vi "Read Props.vi"(8 "error in (no error)":errorcluster, 11 "NumRangeBoolEditorPanel in":refnum<class "NumRangeBoolEditorPanel.lvclass">) -> (0 "error out":errorcluster, 2 "Props":T1, 3 "NumRangeBoolEditorPanel out":refnum<class "NumRangeBoolEditorPanel.lvclass">)   [LabVIEW 2020, in "VolatusGUIControls.lvlib" / "NumRangeBoolEditorPanel.lvclass"]
uses:
  NumRangeBoolEditorPanel.lvclass
  NumRangeBoolEditorPanel.lvclass/NumRangeBoolEditorPanel.ctl
  JSON Props.ctl
  VolatusGUIEditorCore/Label Props.ctl
  VolatusGUIEditorCore/VolatusGUIEditorCore.lvlib
  VolatusGUIEditorCore/Position Props.ctl
  VolatusGUIEditorCore/Boolean Color Props.ctl
  Props.ctl
  VolatusGUIControls.lvlib
  68272f9f-15cf-44f9-b6ab-6d8c4d3063f4.vi
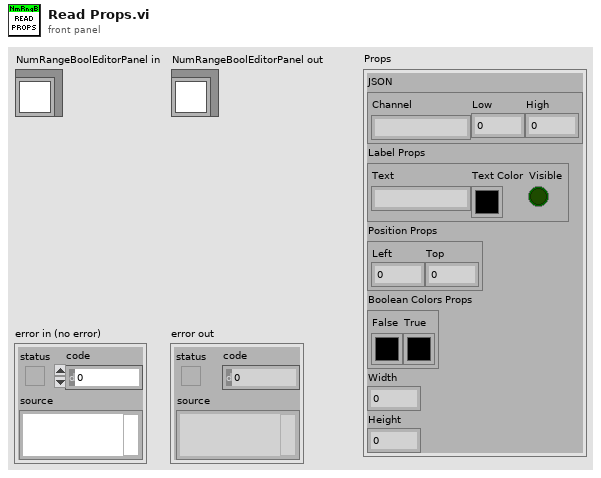
[diagram p1: front panel]
types:
  T1 = typedef "VolatusGUIControls.lvlib/NumRangeBoolEditorPanel.lvclass/Props.ctl" = cluster{"JSON":T2, "Label Props":T3, "Position Props":T4, "Boolean Colors Props":T5, "Width":u16, "Height":u16}
  T2 = typedef "VolatusGUIControls.lvlib/NumRangeBoolEditorPanel.lvclass/JSON Props.ctl" = cluster{"Channel":string, "Low":dbl, "High":dbl}
  T3 = typedef "VolatusGUIEditorCore.lvlib/Label Props.ctl" = cluster{"Text":string, "Text Color":u32, "Visible":bool}
  T4 = typedef "VolatusGUIEditorCore.lvlib/Position Props.ctl" = cluster{"Left":i32, "Top":i32}
  T5 = typedef "VolatusGUIEditorCore.lvlib/Boolean Color Props.ctl" = cluster{"False":u32, "True":u32}
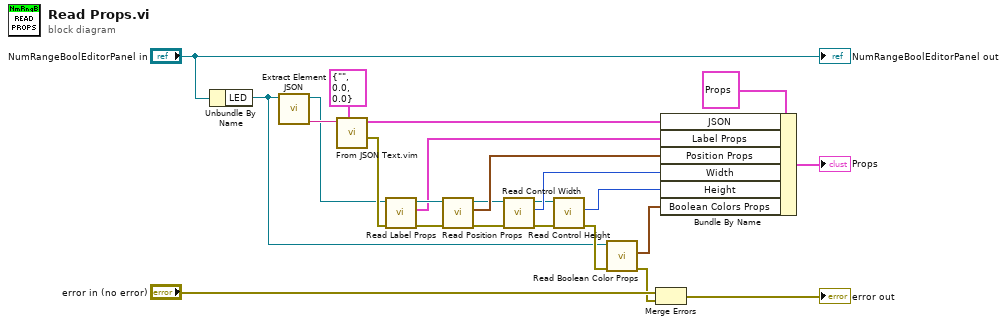
[diagram p0: block diagram]
diagram:
  n1 = Unbundle By Name("NumRangeBoolEditorPanel in") -> ("LED"=w4:refnum<vi>)
  n2 = call "Extract Element JSON.vi"("Ctl Refnum in"=w4) -> ("JSON"=w20:string, "Ctl Refnum"=w16:refnum<vi>)  [unwired: 7 in, 2 out]
  n3 = call "From JSON Text.vim"("Data Type and Default Value"=T2 {"Channel"="", "Low"=0.0, "High"=0.0} ("JSON"), "JSON"=w20) -> ("error out"=w24:errorcluster, "Data out"=w17:T2)  [unwired: 8 in]
  n4 = call "Read Label Props.vi"("error in (no error)"=w24, "Ctl Refnum in"=w16) -> ("error out"=w15:errorcluster, "Label Props"=w13:T3, "Ctl Refnum"=w14:refnum<vi>)  [unwired: 7 in]
  n5 = call "Read Position Props.vi"("error in (no error)"=w15, "Ctl Refnum in"=w14) -> ("error out"=w11:errorcluster, "Position Props"=w12:T4, "Ctl Refnum"=w10:refnum<vi>)  [unwired: 7 in]
  n6 = call "Read Control Width.vi"("error in"=w11, "Control in"=w10) -> ("error out"=w8:errorcluster, "Width"=w9:u32, "Control"=w7:refnum<vi>)  [unwired: 7 in]
  n7 = call "Read Control Height.vi"("error in"=w8, "Control in"=w7) -> ("error out"=w5:errorcluster, "Height"=w6:u32)  [unwired: 7 in, 1 out]
  n8 = call "Read Boolean Color Props.vi"("error in (no error)"=w5, "Control in"=w4) -> ("error out"=w1:errorcluster, "Boolean Colors Props"=w3:T5)  [unwired: 7 in, 1 out]
  n9 = Merge Errors("error in (no error)", w1) -> (→"error out":errorcluster)
  n10 = Bundle By Name(cluster=T1 {"JSON"={"Channel"="", "Low"=0.0, "High"=0.0}, "Label Props"={"Text"="", "Text Color"=0, "Visible"=FALSE}, "Position Props"={"Left"=0, "Top"=0}, "Boolean Colors Props"={"False"=0, "True"=0}, "Width"=0, "Height"=0} ("Props"), "JSON"=w17, "Label Props"=w13, "Position Props"=w12, "Width"=w9, "Height"=w6, "Boolean Colors Props"=w3) -> (→"Props":T1)
  "NumRangeBoolEditorPanel out" <- "NumRangeBoolEditorPanel in"
